vi "AddNewFile.vi"(0 "reference in":refnum<class "Project Panels.lvclass">=refnum, 5 "error in (no error)":errorcluster) -> (14 "reference out":refnum<class "Project Panels.lvclass">, 16 "newData?":bool, 19 "error out":errorcluster={"status"=TRUE, "code"=1556, "source"="G#Object.lvclass:G#Object_NewDebugObject.vi:5270001->Project Panels.lvclass:Project Panels_GetAttributes.vi->Project Panels.lvclass:AddNewFile.vi<ERR>G# Object does not exist. Either it has been destroyed or was never created.\nClass Name: Project Panels\nClass Path: D:\\EOB\\GUI\\Project Panels_class\\Project Panels.lvclass"})   [LabVIEW 2015, in "Project Panels.lvclass"]
uses:
  Project Panels.lvclass
  APP/excelFile_class/fileType.ctl
  SYS/File Controller_llb/File Controller.lvclass
  SYS/Subject Controller_llb/Subject Controller.lvclass
  APP/excelFile_class/excelFile.lvclass
panel:
  in  "Jump Button":bool
  out "String":string="Waiting your decision..."
  in  "File Type:":T1
  in  "File Path Control":path=path "??"
  in  "Open Button":bool
  # "Add Patient/s"
  # "1. Select Path File"
  # "2. Select File Type"
  # "3. Click on the Open\nbutton"
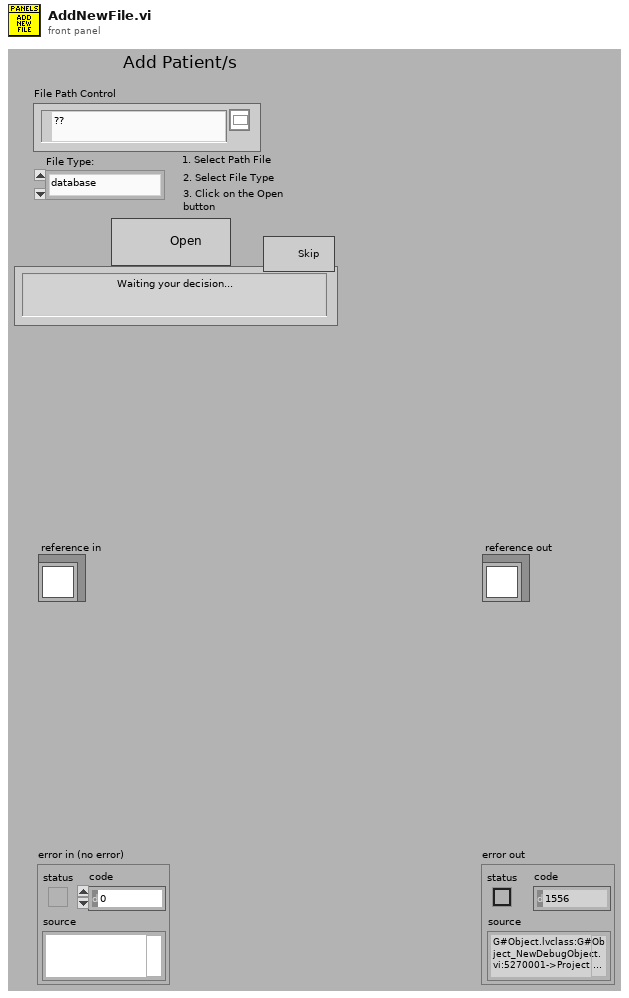
[diagram p1: front panel]
types:
  T1 = typedef "excelFile.lvclass/fileType.ctl" = enum16{"database", "CosmedTest"}
  T2 = typedef "Project Panels.lvclass/ObjectAttributesRef.ctl" = refnum<data-value>
  T3 = typedef "Project Panels.lvclass/ObjectAttributes.ctl" = cluster{"MyAttribute":dbl, "file_controller_ref":refnum<class "File Controller.lvclass">, "subject_controller_ref":refnum<class "Subject Controller.lvclass">}
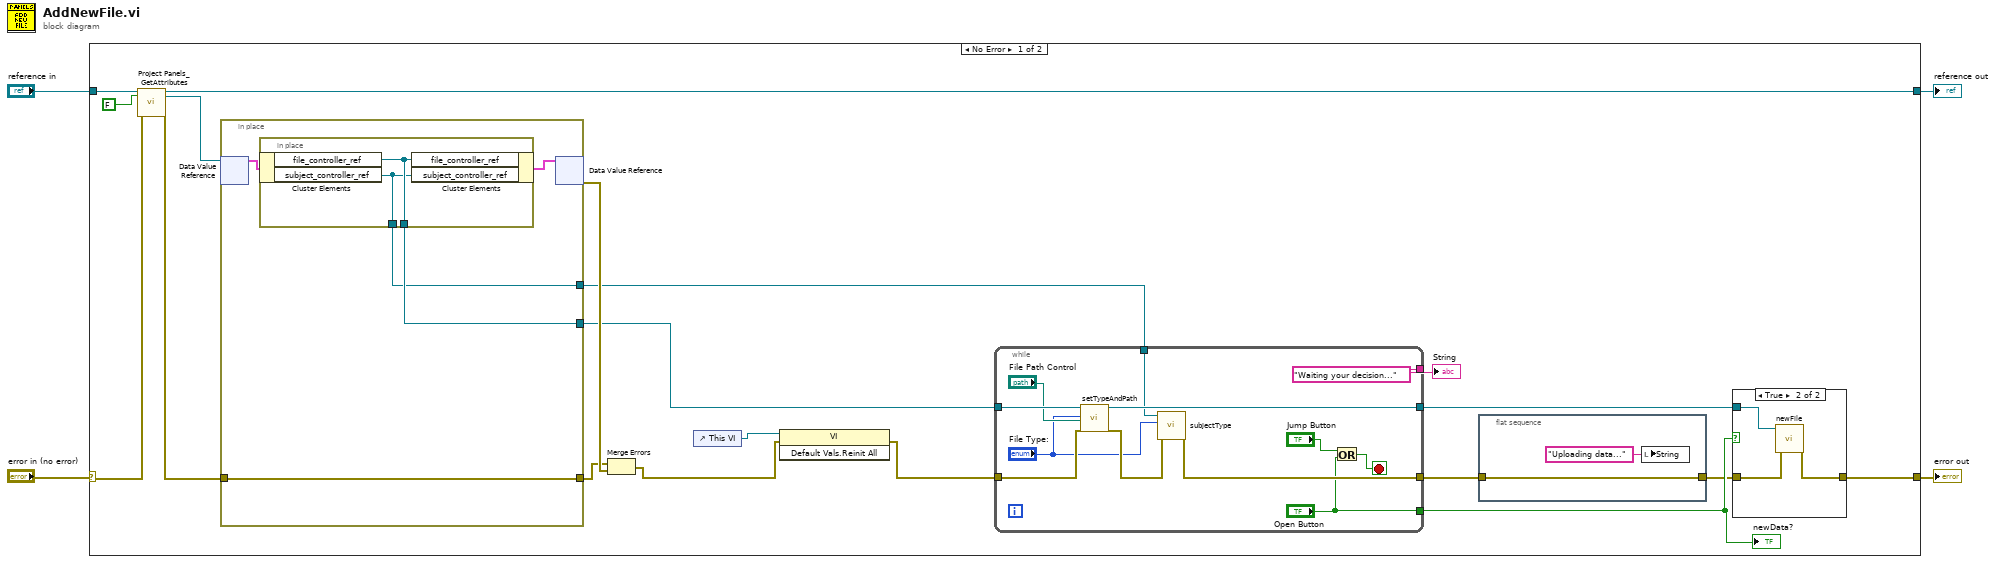
[diagram p0: block diagram]
diagram:
  n1 = case shown="No Error" "error in (no error)" {
    selector: "error in (no error)" -> [w19 w50]
    tunnel: [w12 w50] -> w3
    tunnel: [w17 w49] -> w1
    tunnel: "reference in" -> [w21 w49]
    frame No Error {
      n2 = call "Project Panels_GetAttributes.vi"("reference in"=w21, "return data? (T)"=FALSE, "error in (no error)"=w19) -> ("reference out"=w17:refnum<class "Project Panels.lvclass">, "attributes ref"=w16:T2, "error out"=w18:errorcluster)  [unwired: 13 in, 1 out]
      n3 = in-place {
        in-place-border: w18 -> [w44]
        in-place-border: [w44] -> w22
        in-place-border: [w43] -> w15
        in-place-border: [w42] -> w8
        n4 = in-place-dvr #1(w16) -> (w45:T3)  [unwired: 1 out]
        n5 = in-place {
          in-place-border: [w48] -> w43
          in-place-border: [w47] -> w42
          n6 = in-place-cluster #2(w45) -> ("file_controller_ref"=w48:refnum<class "File Controller.lvclass">, "subject_controller_ref"=w47:refnum<class "Subject Controller.lvclass">)
          n7 = in-place-cluster #2("file_controller_ref"=w48, "subject_controller_ref"=w47) -> (w46:T3)
        }
        n8 = in-place-dvr #1(w46) -> (w23:errorcluster)  [unwired: 1 out]
      }
      n9 = Merge Errors(w22, w23) -> (w10:errorcluster)
      n10 = control-ref of="This VI"() -> (w11:refnum<vi>)
      n11 = invoke class="VI" method="Default Vals.Reinit All"(reference=w11, error in=w10) -> (error out=w9:errorcluster)  [unwired: 1 in, 2 out]
      n12 = while {
        tunnel: w15 -> [w41]
        tunnel: w9 -> [w40]
        tunnel: [w32] -> w6
        tunnel: [w38] -> w14
        tunnel: ["Waiting your decision..."] -> w13
        tunnel: w8 -> [w34]
        tunnel: ["Open Button"] -> w7
        stop <- w36 stop-if-true
        n13 = call "setTypeAndPath.vi"("reference in"=w41, "file_type"="File Type:", "file_path"="File Path Control", "error in (no error)"=w40) -> ("reference out"=w38:refnum<class "File Controller.lvclass">, "error out"=w33:errorcluster)  [unwired: 14 in]
        n14 = call "subjectType.vi"("error in (no error)"=w33, "file_type"="File Type:", "reference in"=w34) -> ("error out"=w32:errorcluster)  [unwired: 7 in, 1 out]
        n15 = Or(x="Jump Button", y="Open Button") -> (x .or. y?=w36:bool)
      }
      "String" <- w13
      "newData?" <- w7
      n16 = flat-sequence {
        tunnel: w6 -> [w25]
        tunnel: [w25] -> w5
        frame #0 {
          n17 = local write "String"("Uploading data..." ("String")) -> ()
        }
      }
      n18 = case shown="True" w7 {
        tunnel: w5 -> [w26 w29]
        tunnel: w14 -> [_ w28]
        tunnel: [w26 w27] -> w12
        frame False {
        }
        frame True {
          n19 = call "newFile.vi"("error in (no error)"=w29, "reference in"=w28) -> ("error out"=w27:errorcluster)  [unwired: 8 in, 1 out]
        }
      }
    }
    frame Error {
    }
  }
  "error out" <- w3
  "reference out" <- w1
